vi "Find All Custom Devices.vi"(8 "error in":errorcluster, 11 "target":refnum<k24>) -> (0 "error out":errorcluster, 2 "custom device refs":T1[](array[typedef]) format="%.0x", 3 "target out":refnum<k24>)   [LabVIEW 2020, in "AIM MIL-STD-1553 Scripting.lvlib"]
doc: "Within the specified target, this VI searches for all the <b>AIM MIL-STD-1553 custom devices</b> and returns all of the references found."
uses:
  AIM MIL-STD-1553 Scripting.lvlib
  NationalInstruments.VeriStand.SystemDefinitionAPI
  <vilib>/NI VeriStand/Custom Device API/Custom Device Item Ref.ctl
  Constants.vi
  <vilib>/NI VeriStand/Custom Device API/Custom Device API.lvlib
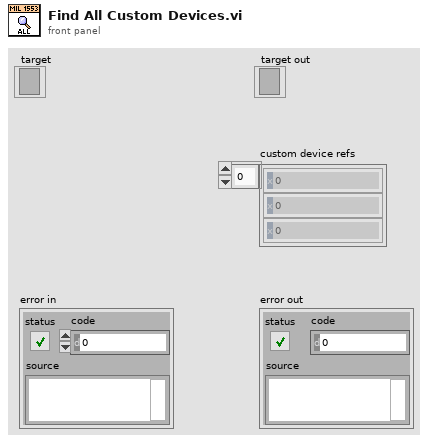
[diagram p1: front panel]
types:
  T1 = typedef "Custom Device API.lvlib/Custom Device Item Ref.ctl" = u64
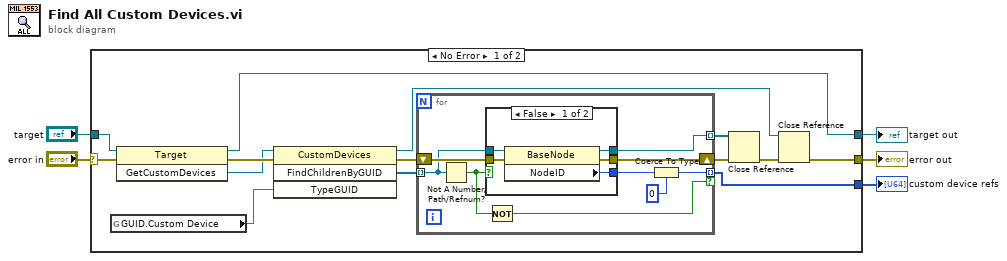
[diagram p0: block diagram]
diagram:
  n1 = case shown="No Error" "error in" {
    selector: "error in" -> [w13 w37]
    tunnel: "target" -> [w15 w36]
    tunnel: [w8 w37] -> w3
    tunnel: [w7 _] -> w1
    tunnel: [w10 w36] -> w2
    frame No Error {
      n2 = global read "Constants.vi" "GUID.Custom Device"() -> (w6:string)
      n3 = invoke on="Invoke Node" class="Target" method="GetCustomDevices"(reference=w15, error in=w13) -> (reference out=w10:refnum<k24>, error out=w19:errorcluster, "GetCustomDevices"=w18:refnum<k24>)  [unwired: 1 in]
      n4 = invoke on="Invoke Node" class="CustomDevices" method="FindChildrenByGUID"(reference=w18, error in=w19, "TypeGUID"=w6) -> (reference out=w11:refnum<k24>, error out=w9:errorcluster, "FindChildrenByGUID"=w14:refnum<k24>[])  [unwired: 1 in, 1 out]
      n5 = for {
        shift-right: [w26] -> w16
        shift-left: w9 -> [w28]
        tunnel: w14 -> [w25] mode=indexing
        tunnel: [w27] -> w17 mode=indexing
        tunnel: [w20] -> w7 mode=indexing if=w23
        n6 = Not A Number/Path/Refnum?(number/path/refnum=w25) -> (NaN/Path/Refnum?=w24:bool)
        n7 = case shown="False" w24 {
          tunnel: [w30 w35] -> w26
          tunnel: w28 -> [w32 w35]
          tunnel: w25 -> [w33 w34]
          tunnel: [w31 w34] -> w27
          tunnel: [w29 _] -> w21
          frame False {
            n8 = property on="Property Node" class="BaseNode"(reference=w33, error in=w32) -> (reference out=w31:refnum<k24>, error out=w30:errorcluster, "NodeID"=w29:u64)
          }
          frame True {
          }
        }
        n9 = Not(x=w24) -> (.not. x?=w23:bool)
        n10 = Coerce To Type(0:w21, 1:T1 0 ("Ballard MIL-STD 1553 custom device")) -> (2:w20:T1)
      }
      n11 = Close Reference(reference=w17, error in (no error)=w16) -> (error out=w12:errorcluster)
      n12 = Close Reference(reference=w11, error in (no error)=w12) -> (error out=w8:errorcluster)
    }
    frame Error {
    }
  }
  "error out" <- w3
  "target out" <- w2
  "custom device refs" <- w1
